vi "insertNewScriptEvent.vi"(6 "delayAll":bool=TRUE, 7 "selectedIndex":i32, 8 "error in (no error)":errorcluster, 9 "index":i32=-1, 10 "ScriptEvent":refnum<class "ScriptEvent.lvclass">, 11 "ScriptEventList in":refnum<class "ScriptEventList.lvclass">) -> (0 "error out":errorcluster, 3 "ScriptEventList out":refnum<class "ScriptEventList.lvclass">)   [LabVIEW 2009, in "Tools.lvlib" / "Scripting.lvlib" / "ScriptEventList.lvclass"]
uses:
  ScriptEventList.lvclass
  ScriptEvent.lvclass
  ScriptEventList.lvclass/ScriptEventList.ctl
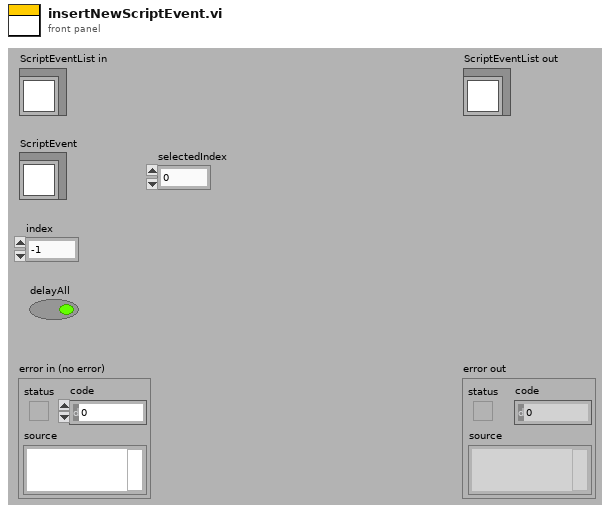
[diagram p1: front panel]
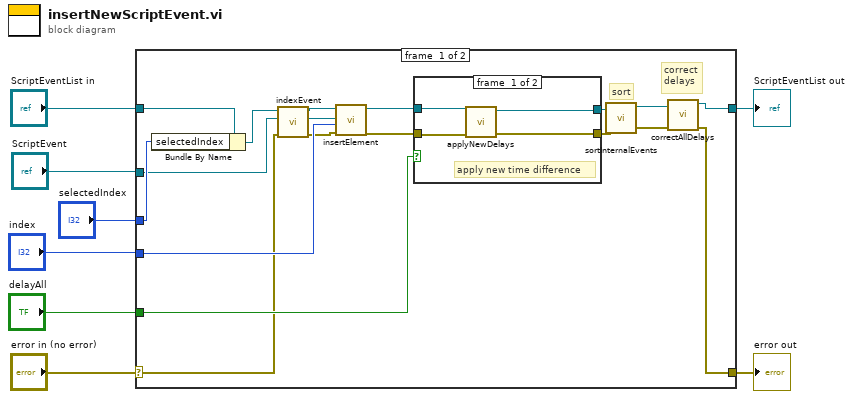
[diagram p0: block diagram]
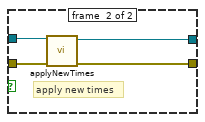
[diagram p2: hidden frame]
diagram:
  n1 = case shown="No Error" "error in (no error)" {
    selector: "error in (no error)" -> [w18 w36]
    tunnel: [w10 w36] -> w7
    tunnel: [w9 w35] -> w5
    tunnel: "ScriptEventList in" -> [w23 w35]
    tunnel: "ScriptEvent" -> [w20 _]
    tunnel: "delayAll" -> [w24 _]
    tunnel: "index" -> [w21 _]
    tunnel: "selectedIndex" -> [w22 _]
    frame #0 {
      # "correct\ndelays"
      # "sort"
      n2 = Bundle By Name(cluster=w23, "selectedIndex"=w22) -> (w15:refnum<class "ScriptEventList.lvclass">)
      n3 = call "indexEvent.vi"("error in (no error)"=w18, "ScriptEvent"=w20, "ScriptEventList in"=w15) -> ("error out"=w19:errorcluster, "ScriptEvent out"=w17:refnum<class "ScriptEvent.lvclass">, "ScriptEventList out"=w16:refnum<class "ScriptEventList.lvclass">)  [unwired: 5 in, 1 out]
      n4 = call "insertElement.vi"("error in (no error)"=w19, "index"=w21, "ScriptEvent"=w17, "ScriptEventList in"=w16) -> ("error out"=w25:errorcluster, "ScriptEventList out"=w26:refnum<class "ScriptEventList.lvclass">)  [unwired: 6 in]
      n5 = case shown="False" w24 {
        tunnel: w26 -> [w30 w34]
        tunnel: w25 -> [w29 w33]
        tunnel: [w28 w32] -> w14
        tunnel: [w27 w31] -> w13
        frame #0 {
          # "apply new time difference"
          n6 = call "applyNewDelays.vi"("error in (no error)"=w29, "ScriptEventList in"=w30) -> ("error out"=w27:errorcluster, "ScriptEventList out"=w28:refnum<class "ScriptEventList.lvclass">)  [unwired: 8 in]
        }
        frame #1 {
          # "apply new times"
          n7 = call "applyNewTimes.vi"("error in (no error)"=w33, "ScriptEventList in"=w34) -> ("error out"=w31:errorcluster, "ScriptEventList out"=w32:refnum<class "ScriptEventList.lvclass">)  [unwired: 8 in]
        }
      }
      n8 = call "sortInternalEvents.vi"("error in (no error)"=w13, "ScriptEventList in"=w14) -> ("error out"=w11:errorcluster, "ScriptEventList out"=w12:refnum<class "ScriptEventList.lvclass">)  [unwired: 8 in]
      n9 = call "correctAllDelays.vi"("error in (no error)"=w11, "ScriptEventList in"=w12) -> ("error out"=w10:errorcluster, "ScriptEventList out"=w9:refnum<class "ScriptEventList.lvclass">)  [unwired: 8 in]
    }
    frame #1 {
    }
  }
  "error out" <- w7
  "ScriptEventList out" <- w5
